vi "CRUD Read All Example.vi"() -> ()   [LabVIEW 2020, in "ORM_Examples.lvlib"]
doc: "This returns the full result set of a query whose WHERE clause is specified as the input. The results are returned as the private data for the bbPlayers class. Note that the BB Players Map class is also needed."
uses:
  ORM_Examples.lvlib
  BB Players Map/BB Players Map.lvclass
  C:/Program Files/National Instruments/LabVIEW 2020/vi.lib/Viviota/shared/ORM.lvlibp/ORM/TypeMap/TypeMap.lvclass
  BB Players/bbPlayers.lvclass
  f1c9faf1-f0a3-46d6-bda1-6eaf119e77ae.vi
  f1c9faf1-f0a3-46d6-bda1-6eaf119e77ae.vi/a9ccc3c9-891a-4d80-8d4f-837bdef88ccd.vi
  f1c9faf1-f0a3-46d6-bda1-6eaf119e77ae.vi/8216614f-f413-45b3-8111-14f8d0271ea5.vi
  f1c9faf1-f0a3-46d6-bda1-6eaf119e77ae.vi/fc6a5c23-d21f-4d2c-895e-66da96fa9491.vi
  f1c9faf1-f0a3-46d6-bda1-6eaf119e77ae.vi/fc6a5c23-d21f-4d2c-895e-66da96fa9491.vi/9d007ba8-e96f-4737-8d8a-6b46cf7f5c4a.vi
  f1c9faf1-f0a3-46d6-bda1-6eaf119e77ae.vi/fc6a5c23-d21f-4d2c-895e-66da96fa9491.vi/050765a8-e5d4-4415-b637-62775228e838.vi
  <vilib>/Viviota/shared/ORM_ADONet.lvlibp/ADOMapper/ADOMapper.lvclass
  C:/Program Files/National Instruments/LabVIEW 2020/vi.lib/Viviota/shared/ORM.lvlibp/ORM/SqlMapper/SqlMapper.lvclass
  <vilib>/Viviota/shared/ORM.lvlibp/ORM/TypeMap/Write Autokey.vi
  <vilib>/Viviota/shared/ORM.lvlibp/ORM/TypeMap/Write Table Name.vi
  <vilib>/Viviota/shared/ORM_DBC_Sqlite.lvlibp/Sqlite Connect.vi
  <vilib>/Utility/error.llb/Error Cluster From Error Code.vi
  <vilib>/Viviota/shared/ORM.lvlibp/ORM/TypeMap/Read TypeMap.vi
  <vilib>/Viviota/shared/ORM.lvlibp/ORM/Query Result/Next.vi
  <vilib>/Viviota/shared/ORM.lvlibp/ORM/TypeMap/ToLabVIEW_Wrap.vi
  <vilib>/Viviota/shared/ORM.lvlibp/ORM/SqlMapper/End Transaction.vi
  <vilib>/Viviota/shared/ORM.lvlibp/ORM/TypeMap/TypeMap.lvclass
  <vilib>/Viviota/shared/ORM.lvlibp/ORM/Query Result/Query Result.lvclass
  ORM_API/ORM_API.lvlib
  <vilib>/Viviota/shared/ORM_ADONet.lvlibp
  <vilib>/Viviota/shared/ORM_DBC_Sqlite.lvlibp/DBC.lvclass
  C:/Program Files/National Instruments/LabVIEW 2020/vi.lib/Viviota/shared/ORM_ADONet.lvlibp/ADOMapper/ADOMapper.lvclass
panel:
  in  "pName":string
  in  "pNum":i32
  out "Results":T1(array[cluster])
  in  "WHERE":string
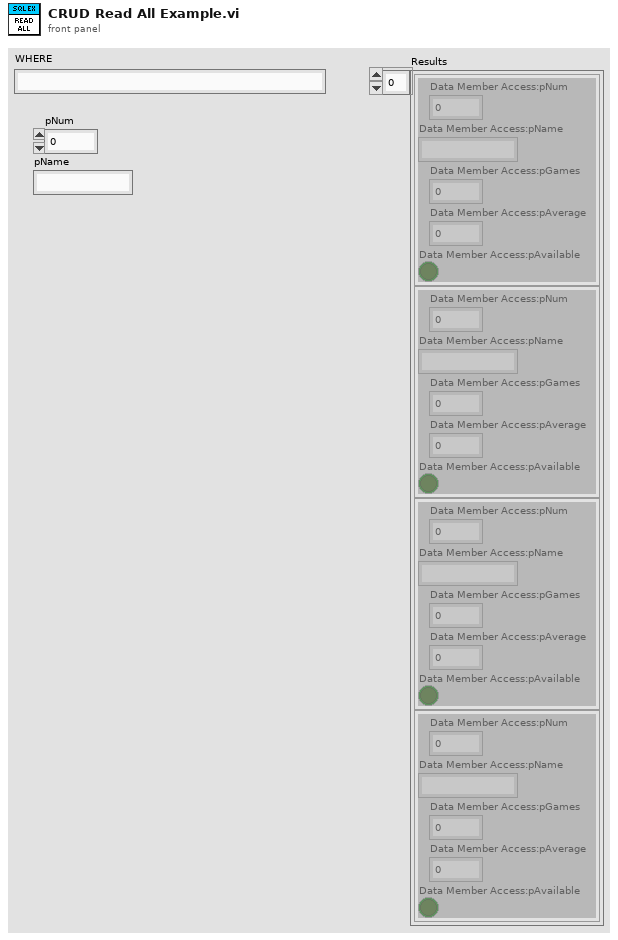
[diagram p1: front panel]
types:
  T1 = cluster{"Data Member Access:pNum":i32, "Data Member Access:pName":string, "Data Member Access:pGames":i32, "Data Member Access:pAverage":dbl, "Data Member Access:pAvailable":bool}[]
  T2 = cluster{"Data Member Access:pNum":i32, "Data Member Access:pName":string, "Data Member Access:pGames":i32, "Data Member Access:pAverage":dbl, "Data Member Access:pAvailable":bool}
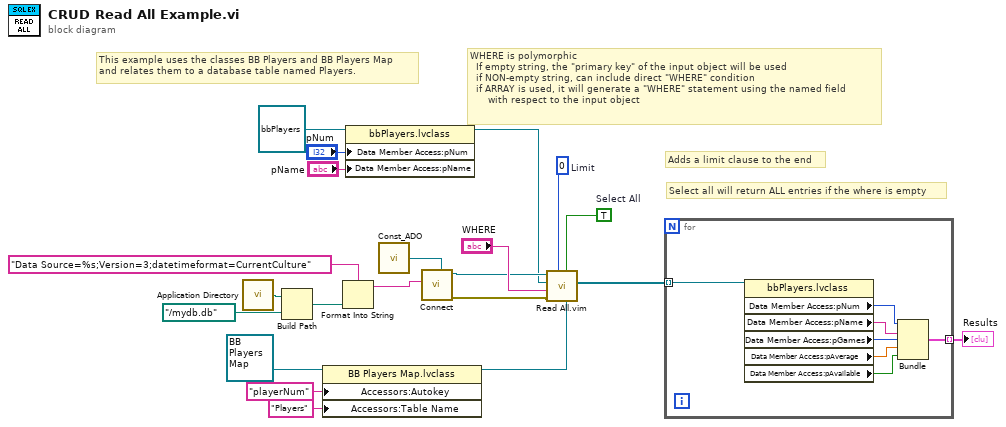
[diagram p0: block diagram]
diagram:
  w1 = i64 0  # Limit
  w5 = TRUE  # Select All
  # "Adds a limit clause to the end"
  # "Select all will return ALL entries if the where is empty"
  # "WHERE is polymorphic\n  If empty string, the \"primary key\" of the input object will be used\n  if NON-empty string, can include direct \"WHERE\" condition\n  if ARRAY is used, it will generate a \"WHERE\" statement using the named field\n      with respect to the input object"
  # "This example uses the classes BB Players and BB Players Map\nand relates them to a database table named Players."
  n1 = call <vilib>:"Application Directory.vi"() -> ("Application Directory"=w12:path)
  n2 = Build Path(base path=w12, name or relative path=path "../mydb.db" ("file out")) -> (appended path=w13:path)
  n3 = property class="BB Players Map.lvclass"(reference=refnum<class "BB Players Map.lvclass"> refnum ("BB Players Map.lvclass"), "Accessors:Autokey"="playerNum" ("Autokey"), "Accessors:Table Name"="Players" ("Table Name")) -> (reference out=w18:refnum<class "BB Players Map.lvclass">)  [unwired: 1 in, 1 out]
  n4 = Format Into String(format string="Data Source=%s;Version=3;datetimeformat=CurrentCulture" ("connectionStringName"), w13) -> (resulting string=w8:string)  [unwired: 2 in, 1 out]
  n5 = property class="bbPlayers.lvclass"(reference=refnum<class "bbPlayers.lvclass"> refnum ("bbPlayers.lvclass"), "Data Member Access:pNum"="pNum", "Data Member Access:pName"="pName") -> (reference out=w4:refnum<class "bbPlayers.lvclass">)  [unwired: 1 in, 1 out]
  n6 = call <vilib>:"Const_ADO.vi"() -> ("ADOMapper"=w9:refnum<class "ADOMapper.lvclass">)
  n7 = call-poly "Connect.vi"("SqlMapper Type"=w9, "Connection String"=w8) -> ("error out"=w6:errorcluster, "SqlMapper out"=w7:refnum<class "ADOMapper.lvclass">)  [unwired: 8 in]
  n8 = call "Read All.vim"("TypeMap in"=w18, "Select All"=w5, "Limit"=w1, "error in (no error)"=w6, "WHERE"="WHERE", "Object"=w4, "SqlMapper in"=w7) -> ("Query Results"=w14:refnum<class "bbPlayers.lvclass">[])  [unwired: 2 in, 2 out]
  n9 = for {
    tunnel: w14 -> [w22] mode=indexing
    tunnel: [w23] -> w17 mode=indexing
    n10 = property class="bbPlayers.lvclass"(reference=w22) -> ("Data Member Access:pNum"=w26:i32, "Data Member Access:pName"=w27:string, "Data Member Access:pGames"=w28:i32, "Data Member Access:pAverage"=w25:dbl, "Data Member Access:pAvailable"=w24:bool)  [unwired: 1 in, 2 out]
    n11 = Bundle("Data Member Access:pNum"=w26, "Data Member Access:pName"=w27, "Data Member Access:pGames"=w28, "Data Member Access:pAverage"=w25, "Data Member Access:pAvailable"=w24) -> (w23:T2)  [unwired: 1 in]
  }
  "Results" <- w17
